vi "shrew Run.vi"(5 "Control":T2(ring), 7 "State":T1, 8 "error in":errorcluster, 10 "Value":variant) -> (0 "error out":errorcluster, 3 "queue out":refnum<queue>)   [LabVIEW 2018]
uses:
  State.ctl
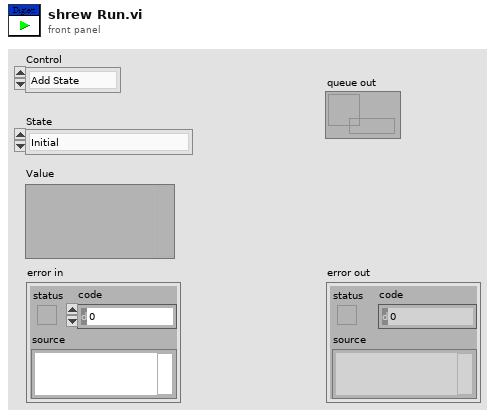
[diagram p1: front panel]
types:
  T1 = typedef "State.ctl" = enum16{"Initial", "Mouse Down", "Random", "Check", "shrew Up", "shrew Down", "shrew Dead", "shrew Wrong", "Exit"}
  T2 = enum16{"Add State", "Insert State", "Initial State", "Release State", "Flush State"}
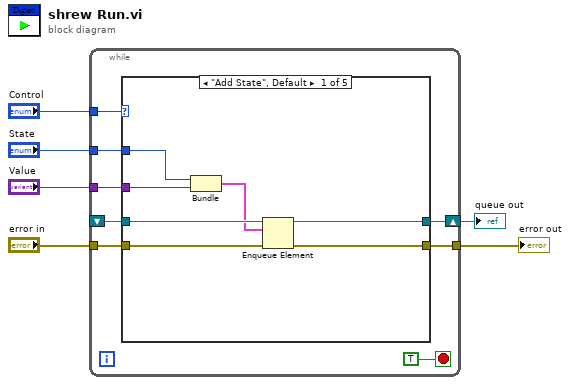
[diagram p0: block diagram]
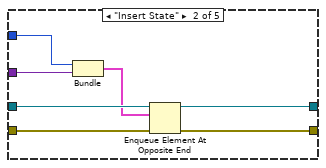
[diagram p2: hidden frame]
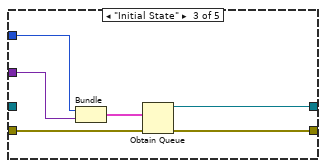
[diagram p3: hidden frame]
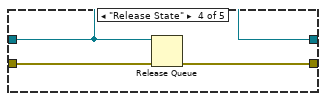
[diagram p4: hidden frame]
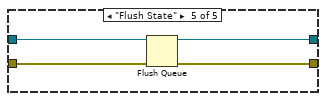
[diagram p5: hidden frame]
diagram:
  n1 = while {
    shift-right: [w8] -> w1
    shift-left: _ -> [w7]
    tunnel: "Control" -> [w14]
    tunnel: "error in" -> [w12]
    tunnel: [w11] -> w4
    tunnel: "State" -> [w10]
    tunnel: "Value" -> [w9]
    stop <- TRUE stop-if-true
    n2 = case shown="\"Add State\", Default" w14 {
      tunnel: w12 -> [w20 w27 w34 w37 w39]
      tunnel: [w19 w26 w33 w36 w38] -> w11
      tunnel: w10 -> [w16 w23 w32 _ _]
      tunnel: w9 -> [w17 w24 w31 _ _]
      tunnel: [w18 w25 w29 w35 w40] -> w8
      tunnel: w7 -> [w21 w28 _ w35 w41]
      frame "Add State", Default {
        n3 = Bundle("State"=w16, "Value"=w17) -> (w15:cluster{"State":T1, "Value":variant})  [unwired: 1 in]
        n4 = Enqueue Element(queue=w21, element=w15, error in (no error)=w20) -> (queue out=w18:refnum<queue>, error out=w19:errorcluster)  [unwired: 1 in, 1 out]
      }
      frame "Insert State" {
        n5 = Bundle("State"=w23, "Value"=w24) -> (w22:cluster{"State":T1, "Value":variant})  [unwired: 1 in]
        n6 = Enqueue Element At Opposite End(queue=w28, element=w22, error in (no error)=w27) -> (queue out=w25:refnum<queue>, error out=w26:errorcluster)  [unwired: 1 in, 1 out]
      }
      frame "Initial State" {
        n7 = Bundle("State"=w32, "Value"=w31) -> (w30:cluster{"State":T1, "Value":variant})  [unwired: 1 in]
        n8 = Obtain Queue(element data type=w30, error in (no error)=w34) -> (queue out=w29:refnum<queue>, error out=w33:errorcluster)  [unwired: 3 in, 1 out]
      }
      frame "Release State" {
        n9 = Release Queue(queue=w35, error in (no error)=w37) -> (error out=w36:errorcluster)  [unwired: 1 in, 2 out]
      }
      frame "Flush State" {
        n10 = Flush Queue(queue=w41, error in (no error)=w39) -> (queue out=w40:refnum<queue>, error out=w38:errorcluster)  [unwired: 1 out]
      }
    }
  }
  "error out" <- w4
  "queue out" <- w1
